vi "DetectLocalCameras.vi"(8 "error in (no error)":errorcluster, 10 "network configuration":T3[](array[typedef]) {"IP Address Request Mode" items=["Static"=1, "DHCP/Link Local"=2, "Link-Local Only"=4, "DHCP Only"=8]; "Adapter Mode" items=["Disabled"=1, "TCP/IP Ethernet"=2, "Deterministic"=4, "EtherCAT"=8, "TCP/IP WLAN Connect"=32, "TCP/IP WLAN Create"=64]}, 11 "config":T1) -> (0 "error out":errorcluster, 1 "new cameras":T2[](array[typedef]), 3 "config out":T1)   [LabVIEW 2017, in "IrManageCameras.lvlib"]
uses:
  <vilib>/addons/InsightCM/Devices/Shared/Ir/IrManageCameras/IrManageCameras.lvlib
  <vilib>/addons/SystemInfoProcess/controls/NetworkAdapterSettings.ctl
  <vilib>/addons/InsightCM/Devices/Shared/Ir/IrManageCameras/controls/camera.ctl
  <vilib>/addons/InsightCM/Devices/Shared/Ir/IrManageCameras/controls/config.ctl
  InsightCM/Devices/WebServices/Ir/DataAccessors/action.ctl
  <vilib>/addons/InsightCM/Utilities/DeviceModelHelpers/DeviceModelHelpers.lvlib
  InsightCM/Devices/WebServices/Ir/DataAccessors/VisionWebServiceData.lvlib
  <vilib>/addons/InsightCM/Utilities/GlobalConfiguration/GlobalConfiguration.lvlib
  <vilib>/addons/SystemInfoProcess/SystemInfoProcess.lvlib
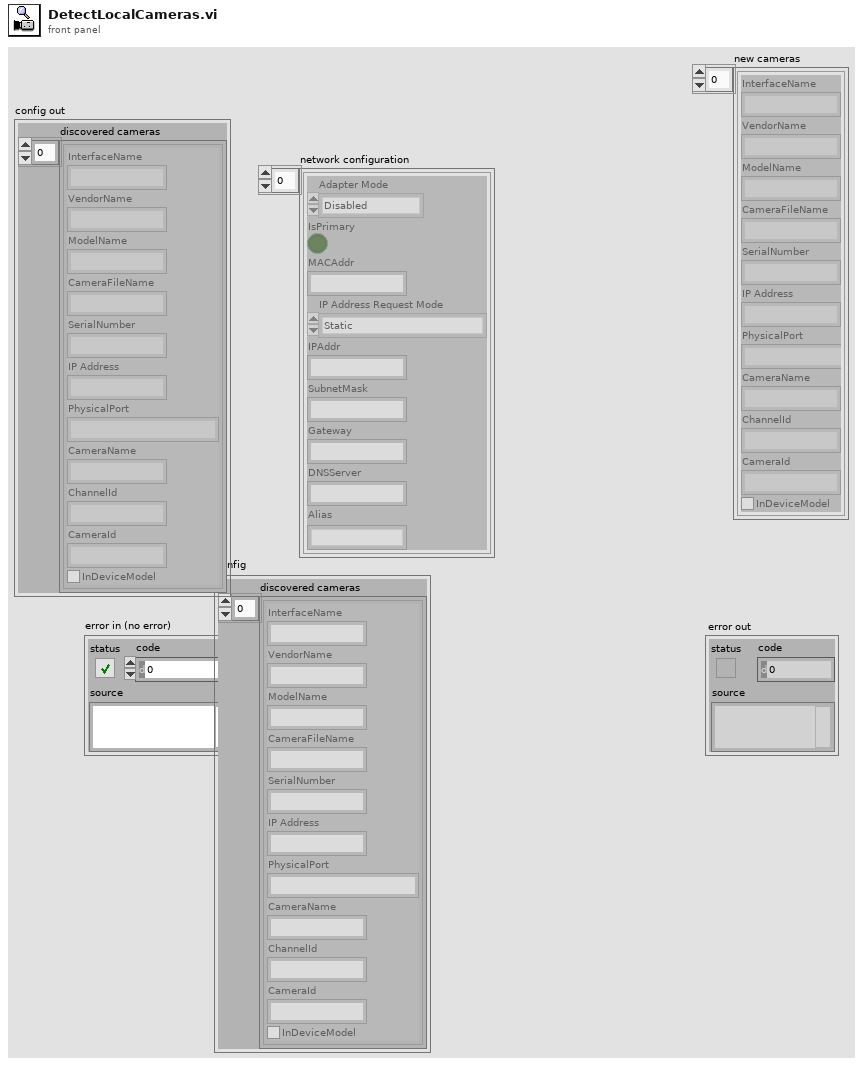
[diagram p1: front panel]
types:
  T1 = typedef "IrManageCameras.lvlib/config.ctl" = cluster{"discovered cameras":T2[]}
  T2 = typedef "IrManageCameras.lvlib/camera.ctl" = cluster{"InterfaceName":string, "VendorName":string, "ModelName":string, "CameraFileName":string, "SerialNumber":string, "IP Address":string, "PhysicalPort":string, "CameraName":string, "ChannelId":string, "CameraId":string, "InDeviceModel":bool}
  T3 = typedef "SystemInfoProcess.lvlib/NetworkAdapterSettings.ctl" = cluster{"Adapter Mode":u32, "IsPrimary":bool, "MACAddr":string, "IP Address Request Mode":u32, "IPAddr":string, "SubnetMask":string, "Gateway":string, "DNSServer":string, "Alias":string}
  T4 = typedef "VisionWebServiceData.lvlib/action.ctl" = enum16{"Get", "Set"}
  T5 = cluster{"Type":u32, "Version":u32, "Flags":u32, "SerialNumberHigh":u32, "SerialNumberLow":u32, "BusType":u32, "InterfaceName":string, "VendorName":string, "ModelName":string, "CameraFileName":string, "CameraAttributeURL":string}[]
  T6 = typedef "R2_Channel.ctl" = cluster{"Id":string, "DeviceId":string, "Name":string, "ChannelType":string, "HardwareKey":string, "HardwareChannel":string, "DataGroup":string, "Keywords":string[], "EquipmentIds":string[], "Properties":T7[], "Metrics":T8[], "AssetNodeId":string, "MeasType":string, "AssetName":string}
  T7 = typedef "KeyValuePair.ctl" = cluster{"Key":string, "Value":string}
  T8 = typedef "Metric.ctl" = cluster{"Id":string, "Name":string, "Unit":string, "Properties":T7[], "MetricDefinitionInstanceId":string}
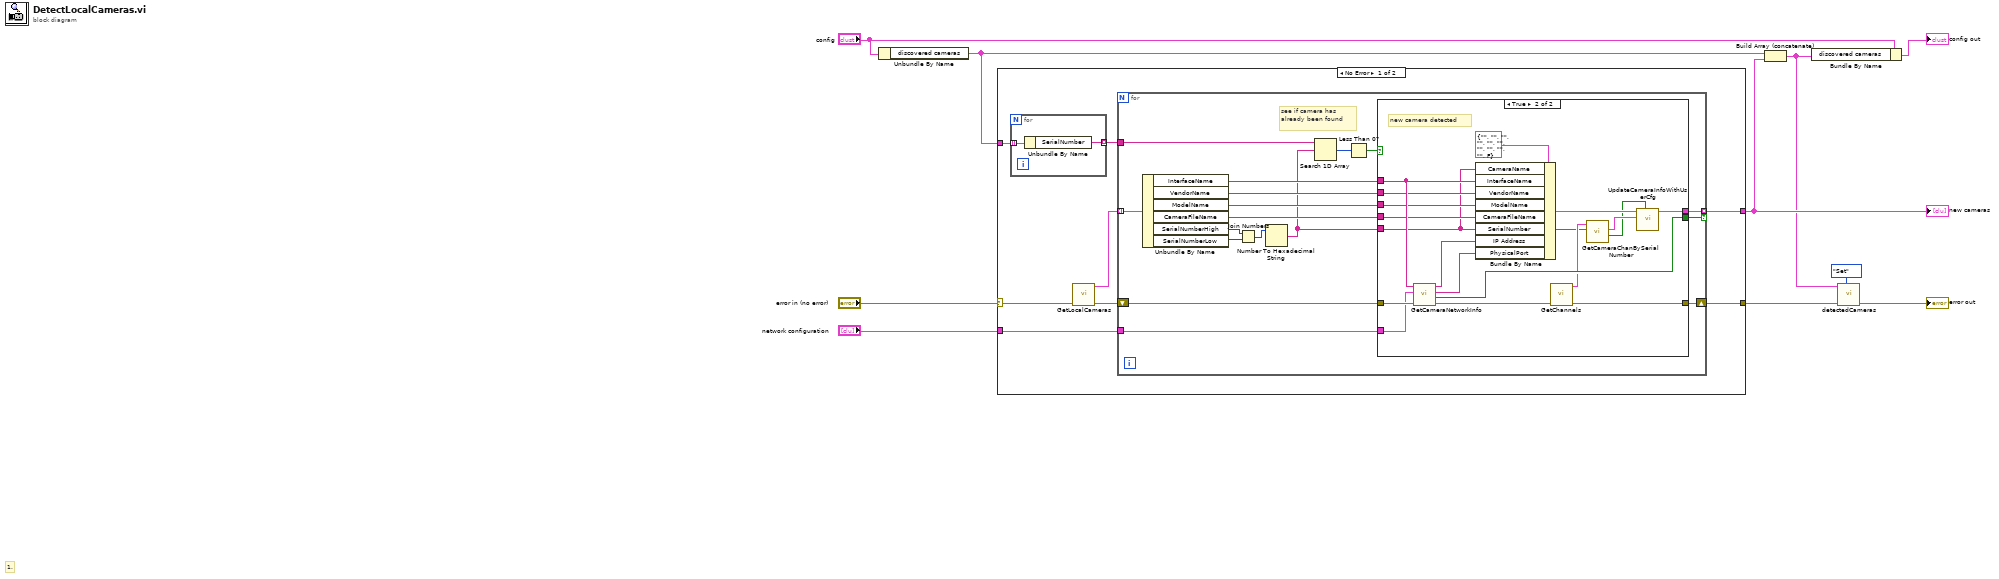
[diagram p0: block diagram]
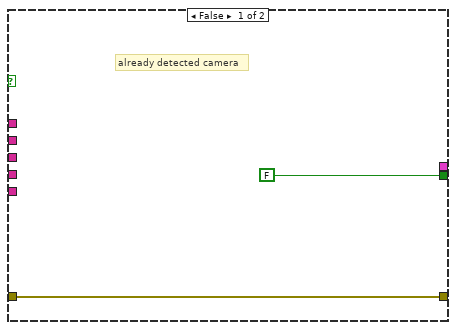
[diagram p2: hidden frame]
diagram:
  # "1."
  n1 = Unbundle By Name("config") -> ("discovered cameras"=w7:T2[])
  n2 = case shown="No Error" "error in (no error)" {
    selector: "error in (no error)" -> [w16 w58]
    tunnel: [w11 w58] -> w3
    tunnel: "network configuration" -> [w17 _]
    tunnel: [w15 _] -> w6
    tunnel: w7 -> [w14 _]
    frame No Error {
      n3 = for {
        tunnel: w14 -> [w57] mode=indexing
        tunnel: [w56] -> w13 mode=indexing
        n4 = Unbundle By Name(w57) -> ("SerialNumber"=w56:string)
      }
      n5 = call <vilib>:"GetLocalCameras.vi"("error in (no error)"=w16) -> ("error out"=w12:errorcluster, "Camera Information Array"=w18:T5)  [unwired: 9 in]
      n6 = for {
        tunnel: w18 -> [w35] mode=indexing
        tunnel: [w30] -> w15 mode=indexing if=w25
        tunnel: w17 -> [w26]
        tunnel: w13 -> [w24]
        shift-right: [w20] -> w11
        shift-left: w12 -> [w19]
        # "see if camera has already been found"
        n7 = Unbundle By Name(w35) -> ("InterfaceName"=w34:string, "VendorName"=w33:string, "ModelName"=w32:string, "CameraFileName"=w31:string, "SerialNumberHigh"=w29:u32, "SerialNumberLow"=w28:u32)
        n8 = Join Numbers(hi=w29, lo=w28) -> ((hi.lo)=w27:u64)
        n9 = Number To Hexadecimal String(2:w27) -> (0:w22:string)  [unwired: 1 in]
        n10 = Search 1D Array(1D array=w24, element=w22) -> (index of element=w23:i32)  [unwired: 1 in]
        n11 = Less Than 0?(x=w23) -> (x < 0?=w21:bool)
        n12 = case shown="True" w21 {
          tunnel: w19 -> [w36 w55]
          tunnel: w34 -> [_ w53]
          tunnel: w33 -> [_ w52]
          tunnel: w32 -> [_ w51]
          tunnel: w31 -> [_ w50]
          tunnel: [_ w46] -> w30
          tunnel: w26 -> [_ w49]
          tunnel: [FALSE w42] -> w25
          tunnel: w22 -> [_ w38]
          tunnel: [w36 w43] -> w20
          frame False {
            # "already detected camera"
          }
          frame True {
            # "new camera detected"
            n13 = call <vilib>:"GetCameraNetworkInfo.vi"("error in (no error)"=w55, "network configuration"=w49, "InterfaceName"=w53) -> ("error out"=w44:errorcluster, "local?"=w42:bool, "Alias"=w48:string, "IPAddress"=w45:string)  [unwired: 5 in]
            n14 = Bundle By Name(cluster=T2 {"InterfaceName"="", "VendorName"="", "ModelName"="", "CameraFileName"="", "SerialNumber"="", "IP Address"="", "PhysicalPort"="", "CameraName"="", "ChannelId"="", "CameraId"="", "InDeviceModel"=FALSE} ("Camera Info"), "CameraName"=w38, "InterfaceName"=w53, "VendorName"=w52, "ModelName"=w51, "CameraFileName"=w50, "SerialNumber"=w38, "IP Address"=w45, "PhysicalPort"=w48) -> (w47:T2)
            n15 = call <vilib>:"GetChannels.vi"("error in (no error)"=w44) -> ("error out"=w43:errorcluster, "channels"=w41:T6[])  [unwired: 8 in, 1 out]
            n16 = call <vilib>:"GetCameraChanBySerialNumber.vi"("camera serial number"=w38, "channels"=w41) -> ("found"=w39:bool, "channel (camera)"=w40:T6)  [unwired: 7 in, 1 out]
            n17 = call <vilib>:"UpdateCameraInfoWithUserCfg.vi"("found"=w39, "channel"=w40, "camera info"=w47) -> ("camera info"=w46:T2)  [unwired: 8 in]
          }
        }
      }
    }
    frame Error {
    }
  }
  "new cameras" <- w6
  n18 = Build Array (concatenate)(w7, w6) -> (w1:T2[])
  n19 = Bundle By Name(cluster="config", "discovered cameras"=w1) -> (→"config out":T1)
  n20 = call "detectedCameras.vi"("action"=action."Set", "error in (no error)"=w3, "Discovered Cameras"=w1) -> ("error out"=→"error out":errorcluster)  [unwired: 7 in, 1 out]
